vi "tcs shm issue Command filter Change Request LV.vi"(8 "error in (no error)":errorcluster, 11 "command_filterChangeRequest_Ctl":cluster{"size":i32, "data":string}) -> (0 "error out":errorcluster, 2 "function return":i32, 3 "command_filterChangeRequest_Ctl out":cluster{"size":i32, "data":string})   [LabVIEW 2016, in "SALLV_tcs.lvlib"]
doc: "int tcs_shm_issueCommand_filterChangeRequestLV(tcs_command_filterChangeRequestLV *command_filterChangeRequest_Ctl );"
uses:
  SALLV_tcs.lvlib
  SALLV_tcs.so
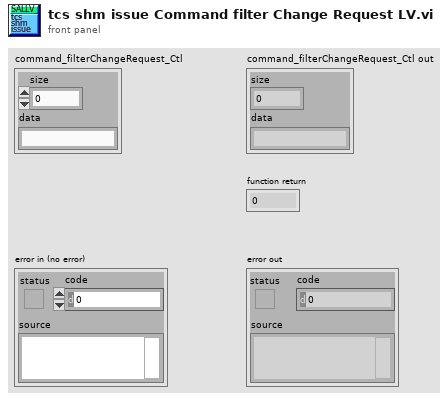
[diagram p1: front panel]
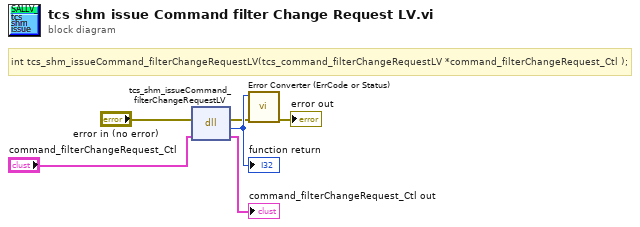
[diagram p0: block diagram]
diagram:
  # "int tcs_shm_issueCommand_filterChangeRequestLV(tcs_command_filterChangeRequestLV *command_filterChangeRequest_Ctl );"
  n1 = dll-call lib="home/andres/Desktop/SALLV_tcs/SALLV_tcs.*" fn="tcs_shm_issueCommand_filterChangeRequestLV"(error in="error in (no error)", "command_filterChangeRequest_Ctl"="command_filterChangeRequest_Ctl") -> (error out=w2:errorcluster, w6:i32, "command_filterChangeRequest_Ctl"=→"command_filterChangeRequest_Ctl out":cluster{"size":i32, "data":string})  [unwired: 2 in, 1 out]
  "function return" <- w6
  n2 = call "Error Converter (ErrCode or Status).vi"("error in (no error)"=w2, "error code"=w6) -> ("error out"=→"error out":errorcluster)  [unwired: 9 in]
